vi "Cleanup.vi"(8 "error in (no error)":errorcluster, 11 "CIFTemplatePlugin in":refnum<class "CIFTemplatePlugin.lvclass">) -> (0 "error out":errorcluster, 3 "CIFTemplatePlugin out":refnum<class "CIFTemplatePlugin.lvclass">)   [LabVIEW 2021, in "CIFTemplatePlugin.lvclass"]
uses:
  CIFTemplatePlugin.lvclass
  CIFTemplatePlugin.lvclass/CIFTemplatePlugin.ctl
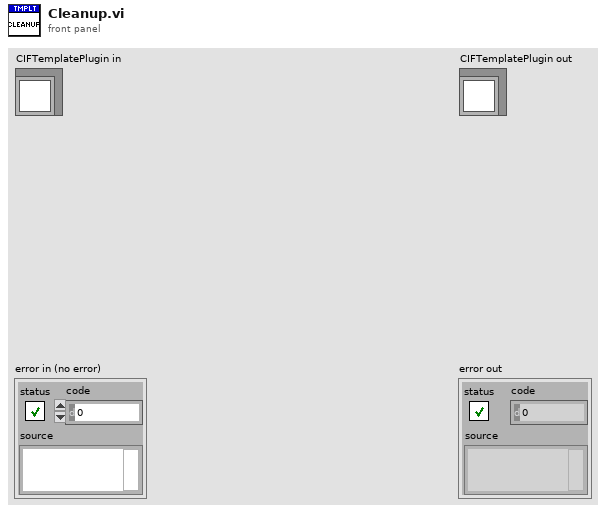
[diagram p1: front panel]
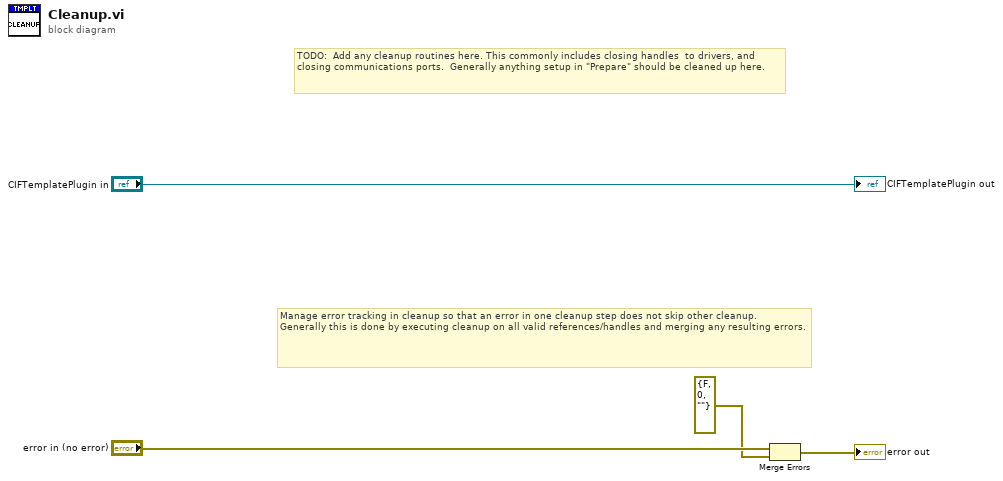
[diagram p0: block diagram]
diagram:
  # "Manage error tracking in cleanup so that an error in one cleanup step does not skip other cleanup.   Generally this is done by executing cleanup on all valid references/handles and merging any resulting errors."
  # "TODO:  Add any cleanup routines here. This commonly includes closing handles  to drivers, and closing communications ports.  Generally anything setup in \"Prepare\" should be cleaned up here."
  n1 = Merge Errors("error in (no error)", errorcluster {"status"=FALSE, "code"=0, "source"=""} ("error in")) -> (→"error out":errorcluster)
  "CIFTemplatePlugin out" <- "CIFTemplatePlugin in"
